vi "激光雷达子VI.vi"(0 "VISA引用句柄输入":refnum<visa-resource-name>, 1 "End Point":dbl=90.0, 2 "Encoding Width":u16, 3 "分割距离阈值":dbl, 4 "拟合度阈值":dbl, 5 "半径下限":dbl, 6 "半径上限":dbl, 7 "错误输入（无错误）":errorcluster, 8 "Start Point":dbl=-90.0, 9 "最少用到的点个数":i32, 10 "Cluster Count":dbl=1.0, 12 "等待时间":u32) -> (18 "最小值距离":dbl, 20 "VISA引用句柄输出":refnum<visa-resource-name>, 21 "最小值角度":dbl, 22 "删除0点个数":u32, 23 "绘图信息":cluster{"X":dbl[], "Y":dbl[]}[](array[cluster]), 24 "拟合结果":T1(array[cluster]), 25 "圆的个数":i32, 27 "错误输出":errorcluster)   [LabVIEW 2016]
uses:
  <vilib>/ptbypt/NI_PtbyPt.lvlib
  Hokuyo URG Series/Hokuyo URG Series.lvlib
panel:
  # "激光雷达子VI程序"
  # "激光雷达调用信息"
  # "拟合阈值"
  # "输出"
  # "测量控制"
  # "说明：该程序通过激光雷\n达寻找并拟合球。在调用\n该程序之前，需要调用激\n光雷达初始化程序。程序\n结束后需要调用激光雷达\n结束程序。绘图直接绘制\nXY图。\n —SEU LabVIEW CLUB"
  # "最近距离与角度"
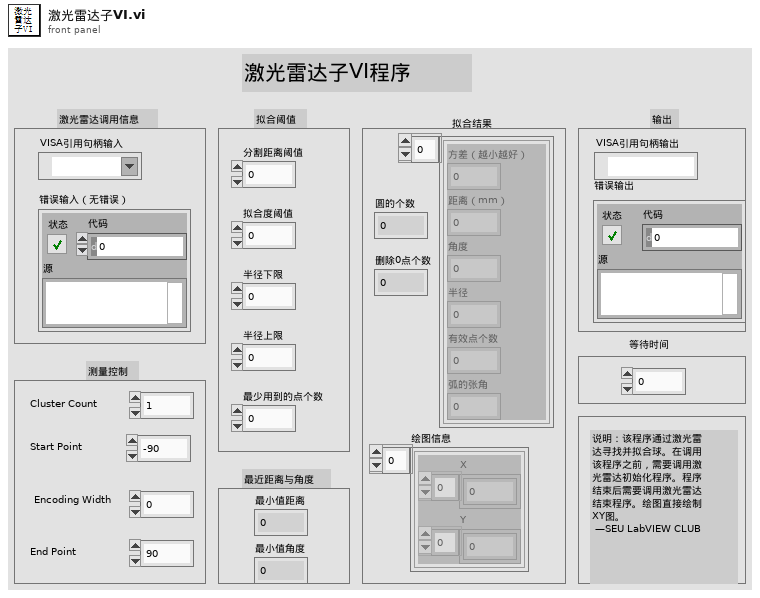
[diagram p1: front panel]
types:
  T1 = cluster{"方差（越小越好）":dbl, "距离（mm）":dbl, "角度":dbl, "半径":dbl, "有效点个数":i32, "弧的张角":dbl}[]
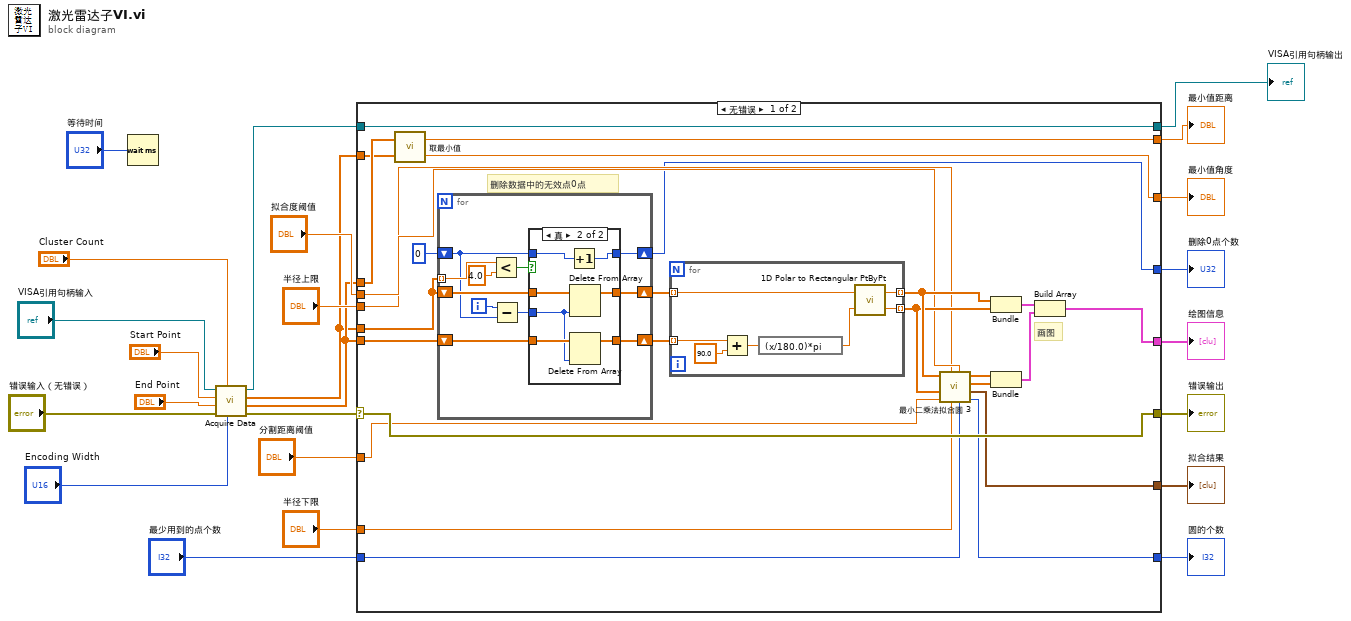
[diagram p0: block diagram]
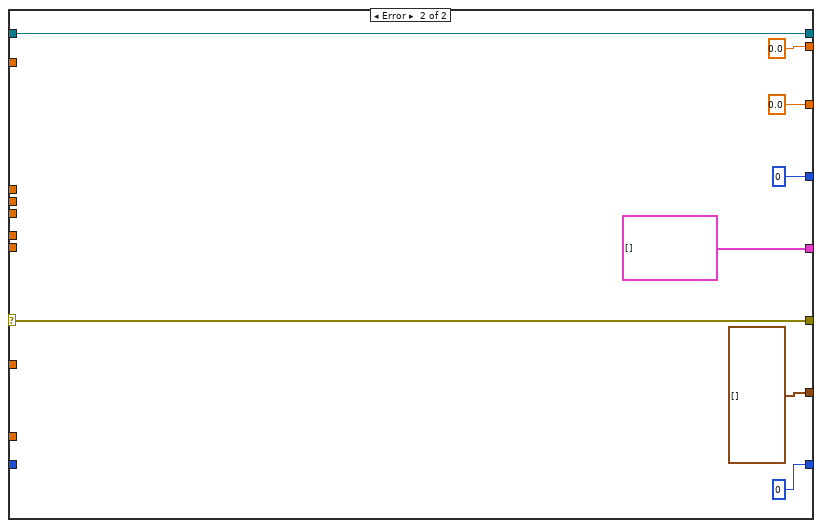
[diagram p3: hidden frame]
diagram:
  n1 = Wait (ms)(milliseconds to wait="等待时间") -> ()  [unwired: 1 out]
  n2 = call "Acquire Data.vi"("Data Encoding Width (3 Byte)"="Encoding Width", "Cluster Count (1)"="Cluster Count", "error in (no error)"="错误输入（无错误）", "End Point (120°)"="End Point", "Start Point (-120°)"="Start Point", "VISA resource name"="VISA引用句柄输入") -> ("error out"=w4:errorcluster, "Direction"=w13:dbl[], "Magnitude"=w12:dbl[], "VISA resource name out"=w3:refnum<visa-resource-name>)  [unwired: 2 in]
  n3 = case shown="无错误" w4 {
    selector: w4 -> [w49 w86]
    tunnel: [w49 w86] -> w1
    tunnel: w3 -> [w50 w85]
    tunnel: [w50 w85] -> w2
    tunnel: w12 -> [w45 _]
    tunnel: w13 -> [w44 _]
    tunnel: w12 -> [w36 _]
    tunnel: w13 -> [w37 _]
    tunnel: "拟合度阈值" -> [w35 _]
    tunnel: "半径上限" -> [w34 _]
    tunnel: "半径下限" -> [w33 _]
    tunnel: "最少用到的点个数" -> [w32 _]
    tunnel: "分割距离阈值" -> [w31 _]
    tunnel: [w30 0.0 ("最小值距离")] -> w19
    tunnel: [w29 0.0 ("最小值角度")] -> w20
    tunnel: [w28 u32 0] -> w21
    tunnel: [w27 cluster{"X":dbl[], "Y":dbl[]}[] []] -> w22
    tunnel: [w26 T1 [] ("拟合结果")] -> w23
    tunnel: [w25 0 ("圆的个数")] -> w24
    frame No Error {
      # "删除数据中的无效点0点"
      # "画图"
      n4 = call "取最小值.vi"("距离"=w36, "角度"=w37) -> ("最小值角度"=w29:dbl, "最小值距离"=w30:dbl)
      n5 = for {
        tunnel: w45 -> [w66] mode=indexing
        shift-right: [w65] -> w41
        shift-left: w45 -> [w64]
        shift-right: [w63] -> w28
        shift-left: u32 0 -> [w61]
        shift-right: [w59] -> w40
        shift-left: w44 -> [w58]
        i -> [w62]
        n6 = Less?(x=w66, y=4.0) -> (x < y?=w68:bool)
        n7 = Subtract(x=w62, y=w61) -> (x-y=w60:u32)
        n8 = case shown="真" w68 {
          tunnel: w58 -> [w69 w75]
          tunnel: w64 -> [w71 w78]
          tunnel: [w71 w77] -> w65
          tunnel: [w70 w76] -> w63
          tunnel: w61 -> [w70 w72]
          tunnel: w60 -> [_ w74]
          tunnel: [w69 w73] -> w59
          frame False {
          }
          frame True {
            n9 = Increment(x=w72) -> (x+1=w76:u32)
            n10 = Delete From Array(array=w78, index=w74) -> (array with subset deleted=w77:dbl[])  [unwired: 1 in, 1 out]
            n11 = Delete From Array(array=w75, index=w74) -> (array with subset deleted=w73:dbl[])  [unwired: 1 in, 1 out]
          }
        }
      }
      n12 = for {
        tunnel: w41 -> [w54] mode=indexing
        tunnel: w40 -> [w57] mode=indexing
        tunnel: [w52] -> w39 mode=indexing
        tunnel: [w51] -> w38 mode=indexing
        n13 = Add(x=w57, y=90.0) -> (x+y=w56:dbl)
        n14 = expression code="(x/180.0)*pi" ("degrees to radians")(w56) -> (w53:dbl)
        n15 = call <vilib>:"1D Polar to Rectangular PtByPt.vi"("phase"=w53, "magnitude"=w54) -> ("y"=w51:dbl, "x"=w52:dbl)
      }
      n16 = call "最小二乘法拟合圆 3.vi"("最少用到的点个数"=w32, "方差阈值"=w35, "半径下限"=w33, "半径上限"=w34, "分割距离阈值"=w31, "y"=w38, "x"=w39) -> ("圆的个数"=w25:i32, "拟合结果"=w26:T1, "Y"=w42:dbl[], "X"=w43:dbl[])  [unwired: 1 in]
      n17 = Bundle(w39, w38) -> (w47:cluster{dbl[], dbl[]})  [unwired: 1 in]
      n18 = Bundle("X"=w43, "Y"=w42) -> (w48:cluster{"X":dbl[], "Y":dbl[]})  [unwired: 1 in]
      n19 = Build Array(w47, w48) -> (w27:cluster{"X":dbl[], "Y":dbl[]}[])
    }
    frame Error {
    }
  }
  "圆的个数" <- w24
  "拟合结果" <- w23
  "绘图信息" <- w22
  "删除0点个数" <- w21
  "最小值角度" <- w20
  "最小值距离" <- w19
  "VISA引用句柄输出" <- w2
  "错误输出" <- w1
